vi "Observe Data.vi"(6 "Time Stamp":timestamp, 8 "error in (no error)":errorcluster, 9 "Value":variant, 10 "Datum Name":string, 11 "ModelCountsObservations in":refnum<class "ModelTimesNObservations.lvclass">) -> (0 "error out":errorcluster, 3 "ModelCountsObservations out":refnum<class "ModelTimesNObservations.lvclass">)   [LabVIEW 2017, in "BenchmarkObservationRate.lvlib" / "ModelTimesNObservations.lvclass"]
doc: "<License>\nCopyright © 2017 Composed Systems, LLC | All rights reserved\nwww.composed.io\n\nAuthor: Ethan Stern <ethan.stern@composed.io>\n\nThis software is provided \"AS IS\" WITHOUT WARRANTIES, either express or implied, AND IS FOR EDUCATIONAL PURPOSES ONLY.\n</License>"
uses:
  ModelTimesNObservations.lvclass
  C:/Program Files (x86)/National Instruments/LabVIEW 2017/vi.lib/ActorFramework/Actor/Actor.lvclass
  ModelTimesNObservations.lvclass/ModelTimesNObservations.ctl
  <vilib>/ActorFramework/Actor/Actor.lvclass/Actor.ctl
  <vilib>/ActorFramework/Message Enqueuer/Message Enqueuer.lvclass/Message Enqueuer.ctl
  <vilib>/ActorFramework/Message Enqueuer/Init from Existing Queue.vi
  <vilib>/ActorFramework/Message Enqueuer/Enqueue.vi
  <vilib>/ActorFramework/Stop Msg/Stop Msg.lvclass
  C:/Program Files (x86)/National Instruments/LabVIEW 2017/vi.lib/ActorFramework/Message/Message.lvclass
  <vilib>/ActorFramework/Message Priority Queue/Priority Enqueue.vi
  <vilib>/ActorFramework/Message Enqueuer/Message Enqueuer.lvclass
  <vilib>/ActorFramework/Actor/Actor.lvclass
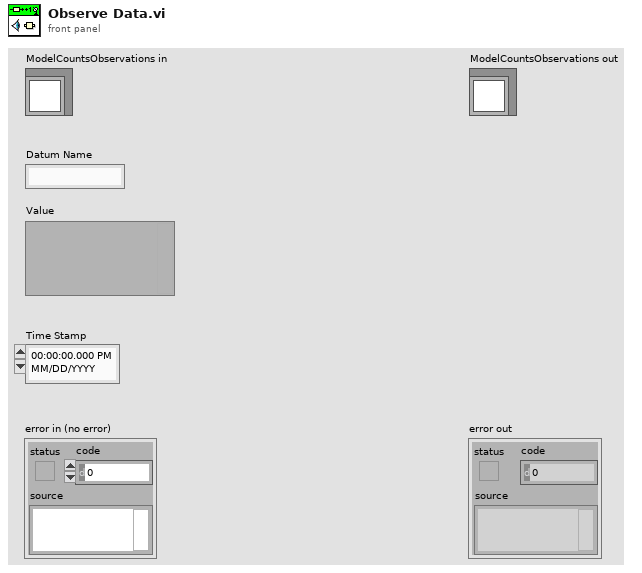
[diagram p1: front panel]
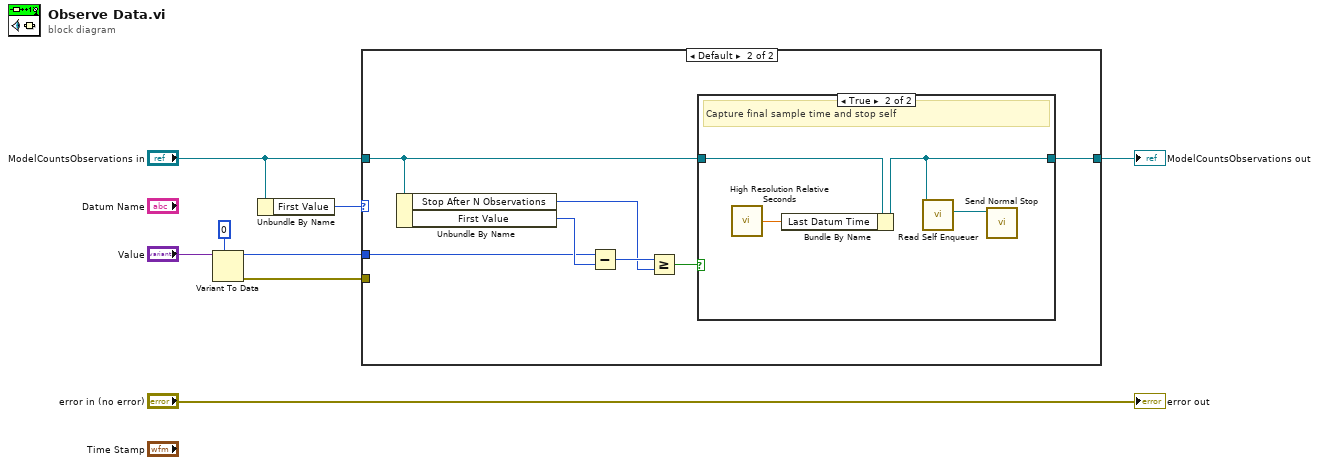
[diagram p0: block diagram]
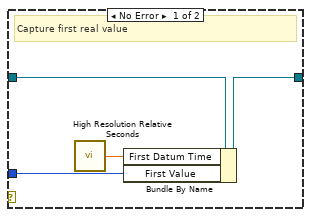
[diagram p3: hidden frame]
diagram:
  n1 = Variant To Data(type=0, Variant="Value") -> (data=w4:i32, error out=w5:errorcluster)  [unwired: 1 in]
  n2 = Unbundle By Name("ModelCountsObservations in") -> ("First Value"=w2:i32)
  n3 = case shown="Default" w2 {
    tunnel: "ModelCountsObservations in" -> [w12 w24]
    tunnel: [w11 w23] -> w6
    tunnel: w5 -> [w10 _]
    tunnel: w4 -> [w9 w20]
    frame -1 {
      n4 = case shown="Error" w10 {
        tunnel: w12 -> [w16 w17]
        tunnel: [w15 w17] -> w11
        tunnel: w9 -> [w13 _]
        frame No Error {
          # "Capture first real value"
          n5 = call <vilib>:"High Resolution Relative Seconds.vi"() -> ("relative seconds"=w14:dbl)
          n6 = Bundle By Name(cluster=w16, "First Datum Time"=w14, "First Value"=w13) -> (w15:refnum<class "ModelTimesNObservations.lvclass">)
        }
        frame Error {
          # "Not a value"
        }
      }
    }
    frame Default {
      n7 = Unbundle By Name(w24) -> ("Stop After N Observations"=w18:i32, "First Value"=w21:i32)
      n8 = Subtract(x=w20, y=w21) -> (x-y=w19:i32)
      n9 = Greater Or Equal?(x=w19, y=w18) -> (x >= y?=w22:bool)
      n10 = case shown="True" w22 {
        tunnel: w24 -> [w25 w29]
        tunnel: [w25 w27] -> w23
        frame False {
        }
        frame True {
          # "Capture final sample time and stop self"
          n11 = call <vilib>:"High Resolution Relative Seconds.vi"() -> ("relative seconds"=w28:dbl)
          n12 = Bundle By Name(cluster=w29, "Last Datum Time"=w28) -> (w27:refnum<class "ModelTimesNObservations.lvclass">)
          n13 = call <vilib>:"Read Self Enqueuer.vi"("Actor"=w27) -> ("Self Enqueuer"=w26:refnum<class "Message Enqueuer.lvclass">)  [unwired: 10 in]
          n14 = call <vilib>:"Send Normal Stop.vi"("Message Enqueuer"=w26) -> ()  [unwired: 10 in, 1 out]
        }
      }
    }
  }
  "ModelCountsObservations out" <- w6
  "error out" <- "error in (no error)"
